vi "ReadAIs.vi"(8 "error in":errorcluster, 10 "Analog Inputs":T1, 11 "VISA resource name":refnum<visa-resource-name>) -> (0 "error out":errorcluster, 2 "Value":u16, 3 "VISA resource name out":refnum<visa-resource-name>)   [LabVIEW 2020, in "HandsOnPi2040.lvlib"]
uses:
  HandsOnPi2040.lvlib
  AnaIns.ctl
  <vilib>/CTI/CTI Visa Drivers/CTI-Visa/CTI-Visa.lvlib
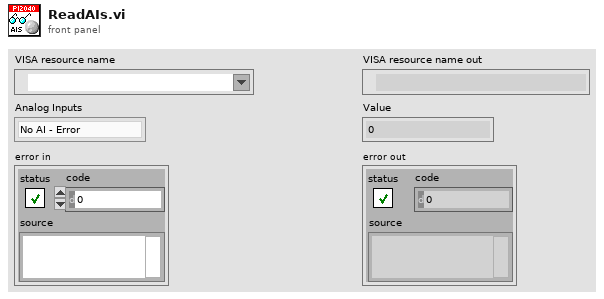
[diagram p1: front panel]
types:
  T1 = typedef "HandsOnPi2040.lvlib/AnaIns.ctl" = enum16{"No AI - Error", "AI1", "AI2"}
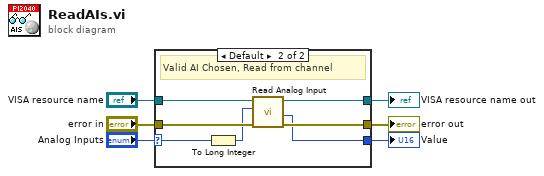
[diagram p0: block diagram]
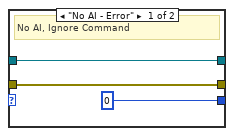
[diagram p2: hidden frame]
diagram:
  n1 = case shown="Default" "Analog Inputs" {
    selector: "Analog Inputs" -> [_ w12]
    tunnel: "VISA resource name" -> [w8 w14]
    tunnel: "error in" -> [w9 w16]
    tunnel: [w8 w13] -> w4
    tunnel: [w9 w15] -> w5
    tunnel: [u16 0 ("Value") w10] -> w1
    frame "No AI - Error" {
      # "No AI, Ignore Command"
    }
    frame Default {
      # "Valid AI Chosen, Read from channel"
      n2 = To Long Integer(number=w12) -> (32bit integer=w11:i32)
      n3 = call <vilib>:"Read Analog Input.vi"("error in (no error)"=w16, "Channel"=w11, "VISA resource name in"=w14) -> ("error out"=w15:errorcluster, "Value"=w10:u16, "VISA resource name"=w13:refnum<visa-resource-name>)  [unwired: 6 in]
    }
  }
  "VISA resource name out" <- w4
  "Value" <- w1
  "error out" <- w5
